vi "[Unguided] Example 2D Array.vi"() -> ()   [LabVIEW 2020]
panel:
  in  "Example 2D Array":i32[][](array[numeric])=[[0, 1, 2, 3, 4, 5, 6, 7, 8, 9], [10, 11, 12, 13, 14, 15, 16, 17, 18, 19], [20, 21, 22, 23, 24, 25, 26, 27, 28, 29], [30, 31, 32, 33, 34, 35, 36, 37, 38, 39]]
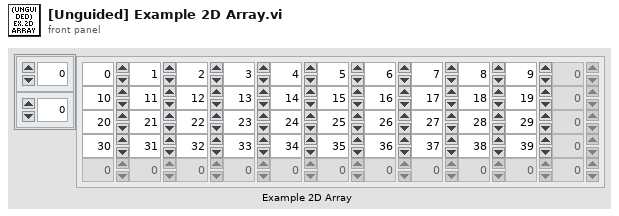
[diagram p1: front panel]
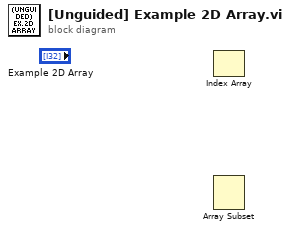
[diagram p0: block diagram]
diagram:
  n1 = Index Array "Index Array"() -> ()  [unwired: 2 in, 1 out]
  n2 = Array Subset "Array Subset"() -> ()  [unwired: 3 in, 1 out]
